vi "LVClass_HasoData Set HasoSlopes.vi"(0 "HasoData":refnum<class "HasoData.lvclass">, 5 "HasoSlopes raw":refnum<class "HasoSlopes.lvclass">, 11 "error in (no error)":errorcluster) -> (4 "HasoData out (dup)":refnum<class "HasoData.lvclass">, 6 "HasoSlopes raw (dup)":refnum<class "HasoSlopes.lvclass">, 15 "error out":errorcluster)   [LabVIEW 2020, in "HasoData.lvclass"]
doc: "Set raw HasoSlopes objects.\n\n--------------------------------------------------------------------------------\n\n<B>HasoDataIn </B> : HasoData object.\n<B>HasoDataOut </B> : HasoData object.\n<B>HasoSlopesRaw </B> : HasoSlopes object.\n<B>ErrorIn </B> : Error\n<B>ErrorOut </B> : Error\n\n--------------------------------------------------------------------------------"
uses:
  HasoData.lvclass
  HasoSlopes.lvclass
  HasoData.lvclass/HasoData.ctl
  LVClass_HasoSlopes Read HasoSlopes _ property.vi
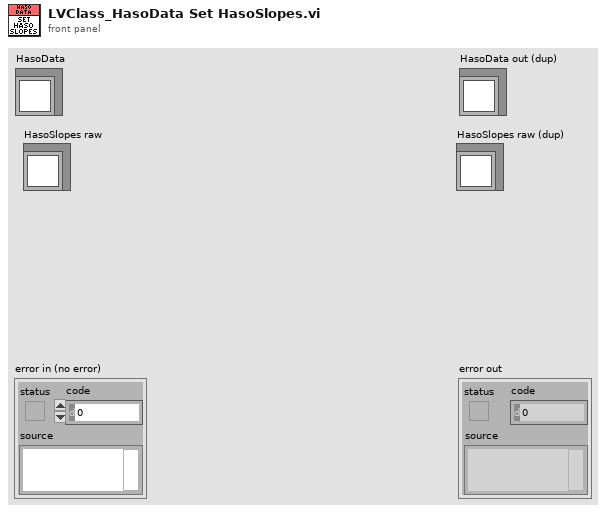
[diagram p1: front panel]
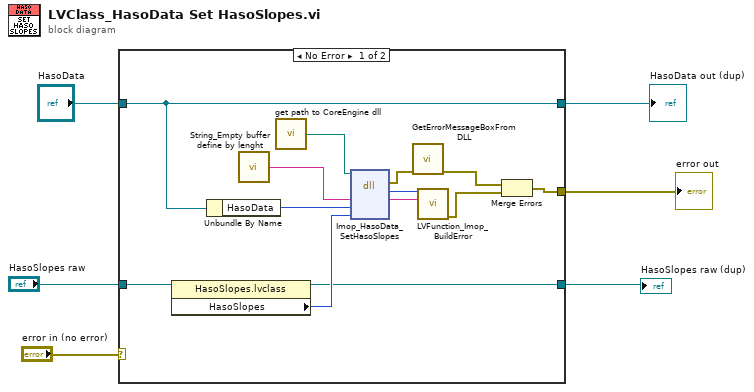
[diagram p0: block diagram]
diagram:
  n1 = case shown="No Error" "error in (no error)" {
    selector: "error in (no error)" -> [_ w22]
    tunnel: [w7 w22] -> w4
    tunnel: [w10 w21] -> w3
    tunnel: "HasoData" -> [w10 w21]
    tunnel: "HasoSlopes raw" -> [w14 w20]
    tunnel: [w12 w20] -> w1
    frame No Error {
      n2 = property class="HasoSlopes.lvclass"(reference=w14) -> (reference out=w12:refnum<class "HasoSlopes.lvclass">, "HasoSlopes"=w13:i32)  [unwired: 1 in, 1 out]
      n3 = Unbundle By Name(w10) -> ("HasoData"=w11:i32)
      n4 = call "String_Empty buffer define by lenght.vi"() -> ("Empty buffer"=w17:string)  [unwired: 1 in]
      n5 = call "get path to CoreEngine dll.vi"() -> ("path to c_interface_vc100.dll"=w16:path)  [unwired: 12 in, 3 out]
      n6 = dll-call lib="D:/2_trunk/Soft_haso/ImOpCoreEngine4_LV2011/DLLs/ImopEngine4_vc100.dll" fn="Imop_HasoData_SetHasoSlopes"(path in=w16, "message"=w17, "objet"=w11, "HasoSlopesRaw"=w13) -> (error out=w15:errorcluster, "return type"=w19:i32, "message"=w18:string)  [unwired: 4 in, 1 out]
      n7 = call "GetErrorMessageBoxFromDLL.vi"("error IN"=w15) -> ("error OUT"=w9:errorcluster)  [unwired: 10 in]
      n8 = call "LVFunction_Imop_BuildError.vi"("code"=w19, "String to Prepend to source (\"\")"=w18) -> ("error out"=w8:errorcluster)  [unwired: 13 in]
      n9 = Merge Errors(w9, w8) -> (w7:errorcluster)
    }
    frame Error {
    }
  }
  "error out" <- w4
  "HasoData out (dup)" <- w3
  "HasoSlopes raw (dup)" <- w1
